vi "var_perm-mode_current-value.vi"() -> ()   [LabVIEW 2010]
panel:
  out "changing mode":bool
  out "in perm mode?":bool
  in  "permanent mode field":dbl
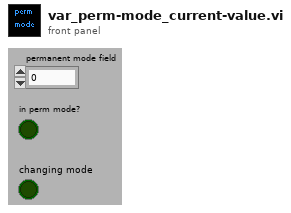
[diagram p1: front panel]
diagram:
